vi "CLT_RunStateMach.vi"(6 "Test Index":i32, 7 "FullConfig":T6={"Bench Params"={"Relative Root Name"="", "Values"={"Step Levels"=0.0, "Resistor Tolerence"=0.0, "Sample Rate"=0.0, "Resistor"=0.0, "Wait Time"=0.0}, "Report Template path"=path "$ReportFiles/ReportTemplate_03.xlsx", "Test Type"="", "Config File Name"="", "Config 2 Use"="", "Skip Pre Lube"=FALSE}, "Test Params"=[], "Pump Params"={"Empty Inches"=0.0, "Full Inches"=0.0, "RNG_SLOW"=0.0, "RNG_CREEP"=0.0, "RNG_STOP "=0.0, "VISA resource name"="", "SPD_SLOW"=0, "SPD_CREEP"=0, "SPD_FAST"=0, "Zero template"=path "", "zero  Settle sec"=0, "Laser Slope"=0.0, "Laser Offset"=0.0, "Sim Fill Rate"=0.0, "Cal Date"="", "Cal Technician"=""}, "DataQ Params"={"Visa Name"="", "Num Chan"=0, "Cal Coef"=[], "Scale "=0, "Cal Date"="", "Cal Technicain"=""}, "Pump Control Ref"={"Fill "=refnum, "Drain"=refnum, "Level PV"=refnum, "Pump Speed"=refnum, "Run Test"=refnum, "Sim"=refnum, "Jog"=refnum, "Level SP"=refnum}, "Bench Status"={"Pump Status"=refnum, "Dataq Status"=refnum, "LaserStatus"=refnum, "ChA Ohms"=refnum, "ChB Ohms"=refnum}} {"Pump Params"."Sim Fill Rate" format="%.3f"; "Pump Params"."Laser Offset" format="%.3f"; "Pump Params"."Laser Slope" format="%.3f"; "Pump Params"."RNG_STOP" format="%#_13g"; "Pump Params"."RNG_CREEP" format="%#_13g"; "Pump Params"."RNG_SLOW" format="%#_13g"}, 11 "TEST State In":T5) -> (1 "Enable":bool, 2 "Level S":dbl, 3 "TEST State Out":T5, 4 "Test Index Out":i32, 5 "Specs Out":T1)   [LabVIEW 2024]
doc: "The \"Run Test\" button selects between MANUAL adjustment of Set Point (SP) by the user or AUTO mode, where:\n1. Start, initial state drains until the tank is empty\n2. Filling, Auto set of SP to Max Fill Inches (or recipie)\n3. FULL Pause when full\n4. Draining Auto set of SP to 0 (or recipie)\n5. EMPTY Paue when empty\n6. Done SP set to 0."
uses:
  Control Definitions/DEF_FullConfig.ctl
  Control Definitions/DEF_BenchParams.ctl
  Control Definitions/DEF_PumpParams.ctl
  Control Definitions/DEF_DataqParams.ctl
  Control Definitions/DEF_PumpCtlRefs.ctl
  Control Definitions/Def_PumpSpeed.ctl
  Control Definitions/DEF_BenchStatus.ctl
  Control Definitions/Def TestState.ctl
  Control Definitions/DEF_SpecsOut.ctl
  Control Definitions/Def Spec RNG.ctl
  Control Definitions/Ded LUT_Status.ctl
  Control Definitions/Global 2.vi
panel:
  out "Timer":dbl
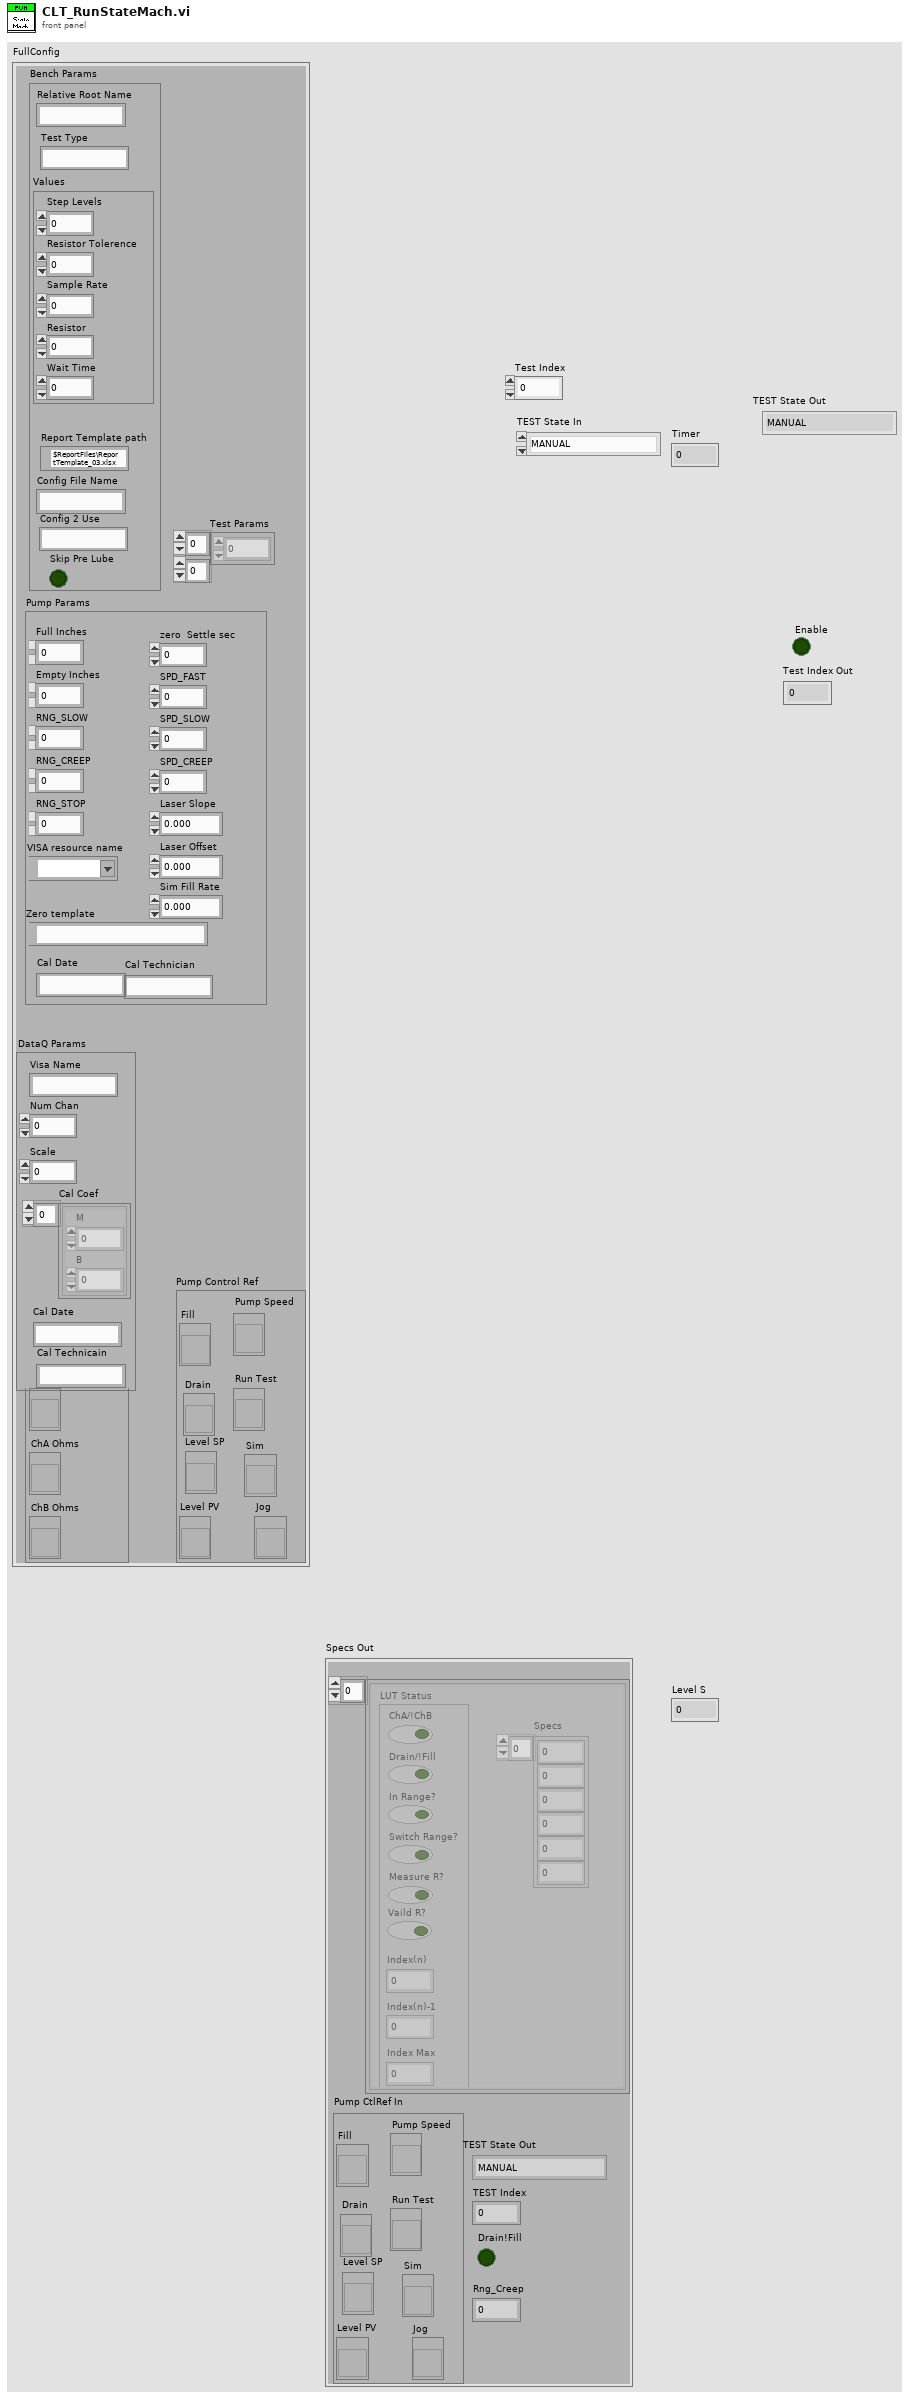
[diagram p1: front panel]
types:
  T1 = typedef "DEF_SpecsOut.ctl" = cluster{"aSpecsTable":T2[], "Pump CtlRef In":T4, "TEST State Out":T5, "TEST Index":i32, "Drain!Fill":bool, "Rng_Creep":dbl}
  T2 = typedef "Def Spec RNG.ctl" = cluster{"Specs":dbl[], "LUT Status":T3}
  T3 = typedef "Ded LUT_Status.ctl" = cluster{"ChA/!ChB":bool, "Drain/!Fill":bool, "In Range?":bool, "Switch Range?":bool, "Measure R?":bool, "Vaild R?":bool, "Index(n)":i32, "Index(n)-1":i32, "Index Max":i32, "Index(n-1)":i32}
  T4 = typedef "DEF_PumpCtlRefs.ctl" = cluster{"Fill ":refnum<vi>, "Drain":refnum<vi>, "Level PV":refnum<vi>, "Pump Speed":refnum<vi>, "Run Test":refnum<vi>, "Sim":refnum<vi>, "Jog":refnum<vi>, "Level SP":refnum<vi>}
  T5 = typedef "Def TestState.ctl" = enum16{"MANUAL", "Start", "Pre-Fill", "Pre-Fill Measure", "Pre-Drain", "Pre-Drain Measure", "Init-Record", "Load Fill Spec", "Filling Hi", "Wait1", "Record Fill", "Load Drain Spec", "Draining Lo", "Wait2", "Record Drain", "Empty", "Done"}
  T6 = typedef "DEF_FullConfig.ctl" = cluster{"Bench Params":T7, "Test Params":dbl[][], "Pump Params":T8, "DataQ Params":T9, "Pump Control Ref":T4, "Bench Status":T10}
  T7 = typedef "DEF_BenchParams.ctl" = cluster{"Relative Root Name":string, "Values":cluster{"Step Levels":dbl, "Resistor Tolerence":dbl, "Sample Rate":dbl, "Resistor":dbl, "Wait Time":dbl}, "Report Template path":path, "Test Type":string, "Config File Name":string, "Config 2 Use":string, "Skip Pre Lube":bool}
  T8 = typedef "DEF_PumpParams.ctl" = cluster{"Empty Inches":dbl, "Full Inches":dbl, "RNG_SLOW":dbl, "RNG_CREEP":dbl, "RNG_STOP ":dbl, "VISA resource name":refnum<visa-resource-name>, "SPD_SLOW":i32, "SPD_CREEP":i32, "SPD_FAST":i32, "Zero template":path, "zero  Settle sec":i32, "Laser Slope":sgl, "Laser Offset":sgl, "Sim Fill Rate":sgl, "Cal Date":string, "Cal Technician":string}
  T9 = typedef "DEF_DataqParams.ctl" = cluster{"Visa Name":string, "Num Chan":i32, "Cal Coef":cluster{"M":dbl, "B":dbl}[], "Scale ":i32, "Cal Date":string, "Cal Technicain":string}
  T10 = typedef "DEF_BenchStatus.ctl" = cluster{"Pump Status":refnum<vi>, "Dataq Status":refnum<vi>, "LaserStatus":refnum<vi>, "ChA Ohms":refnum<vi>, "ChB Ohms":refnum<vi>}
  T11 = typedef "Def_PumpSpeed.ctl" = enum16{"FAST", "SLOW", "CREEP", "STOP"}
  T12 = enum16{"MANUAL", "Start", "Filling", "FULL", "Draining", "EMPTY", "Done"}
  T13 = cluster{"Spec RNG Out":T2[], "Pump Control Ref":T4, "TEST State Out":u16, "Index":i32, bool, "RNG_CREEP":dbl}
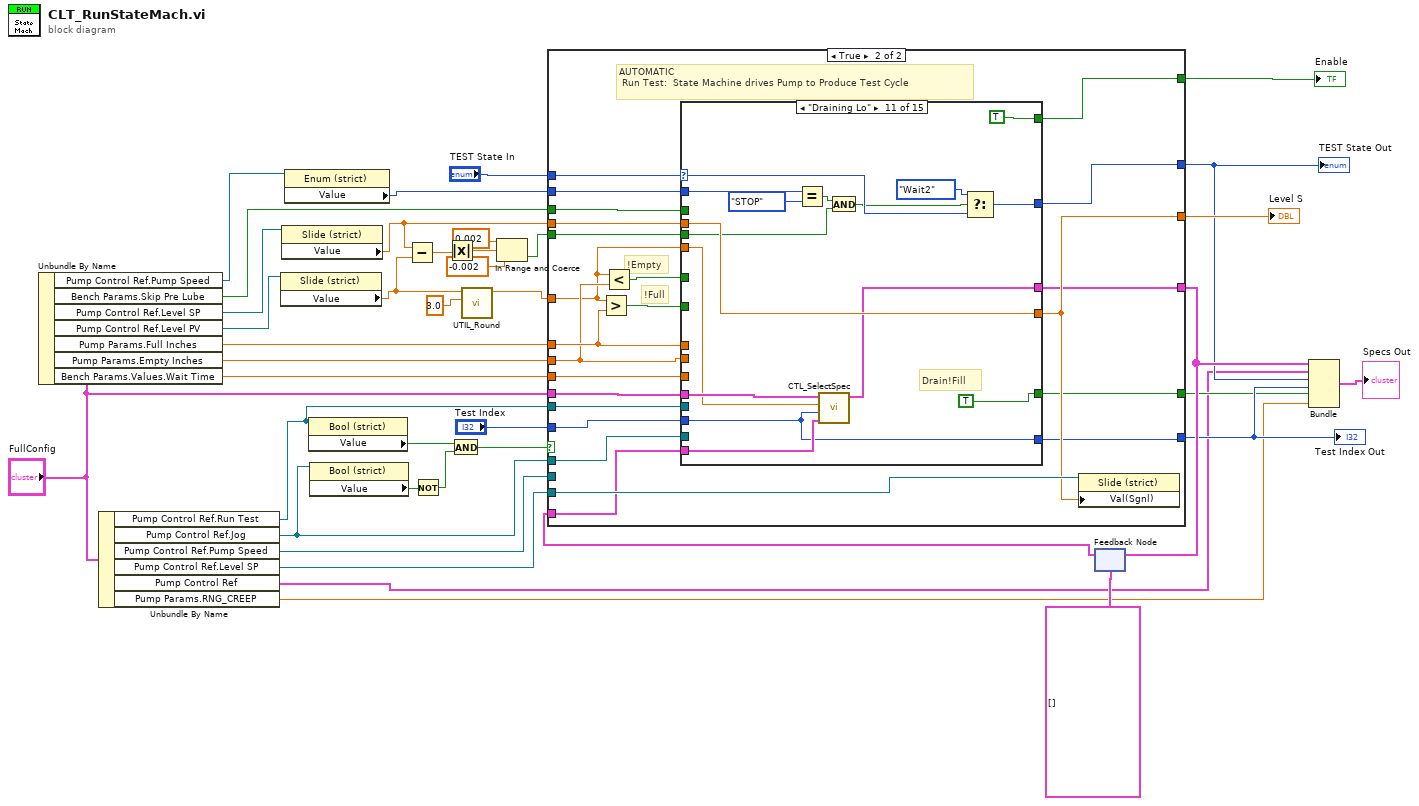
[diagram p0: block diagram]
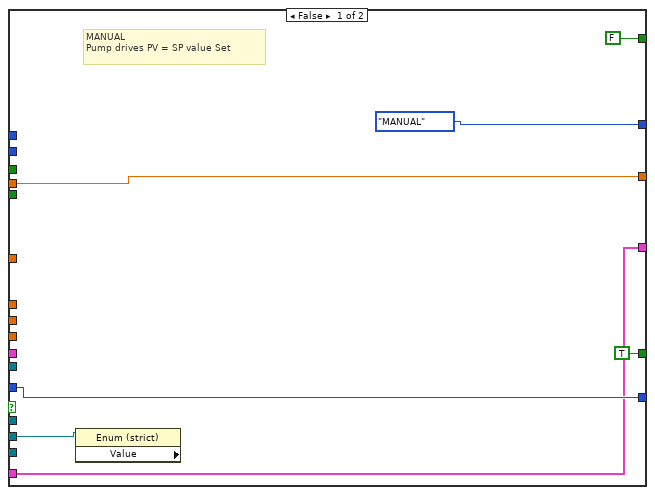
[diagram p2: hidden frame]
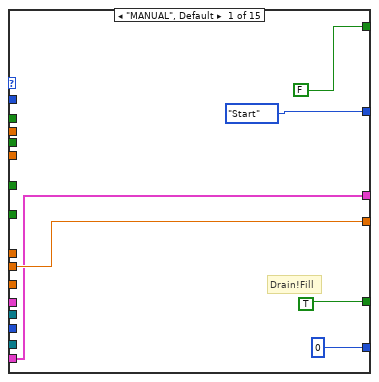
[diagram p3: hidden frame]
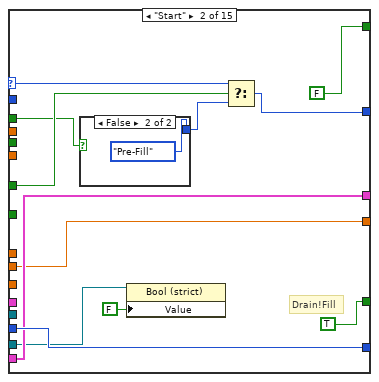
[diagram p4: hidden frame]
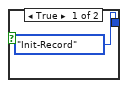
[diagram p5: hidden frame]
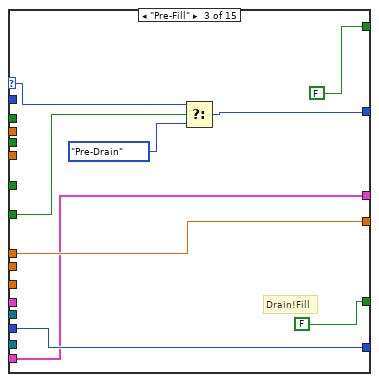
[diagram p6: hidden frame]
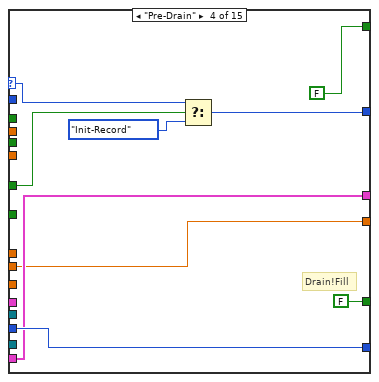
[diagram p7: hidden frame]
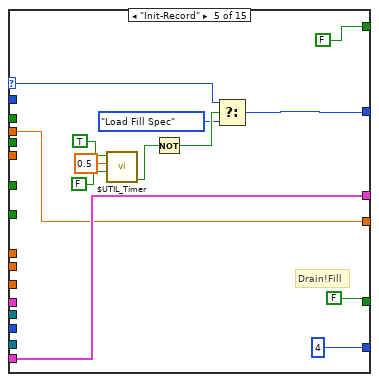
[diagram p8: hidden frame]
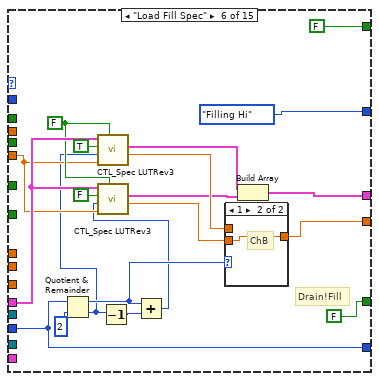
[diagram p9: hidden frame]
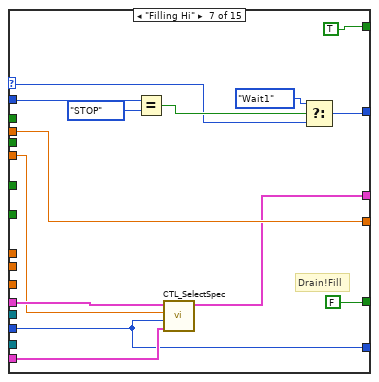
[diagram p11: hidden frame]
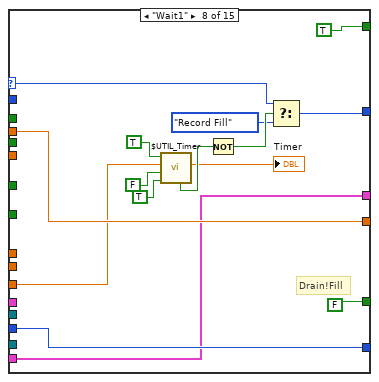
[diagram p12: hidden frame]
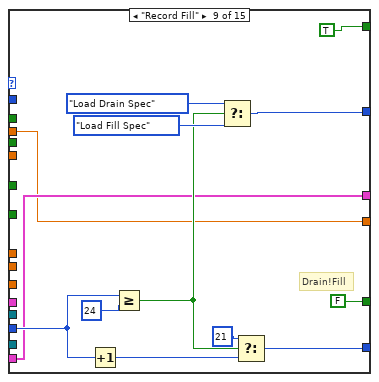
[diagram p13: hidden frame]
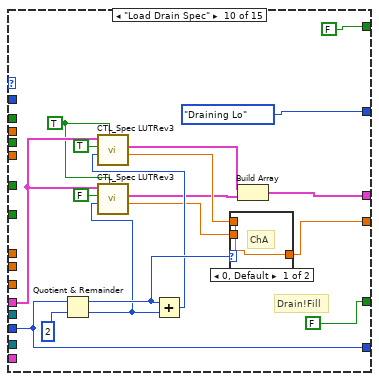
[diagram p14: hidden frame]
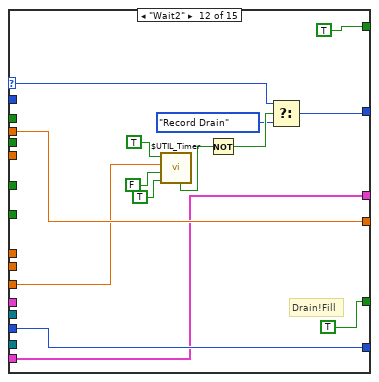
[diagram p16: hidden frame]
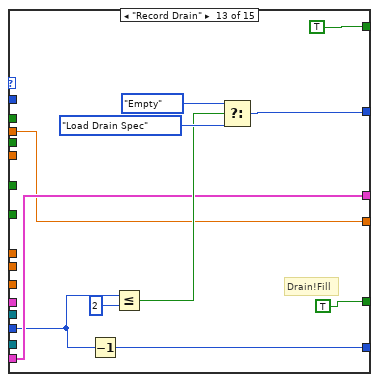
[diagram p17: hidden frame]
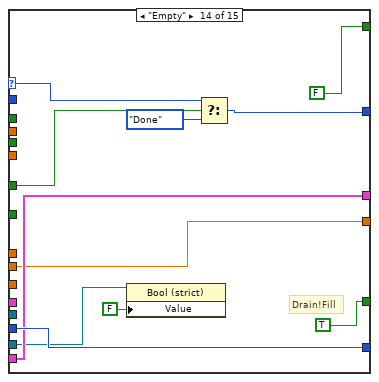
[diagram p18: hidden frame]
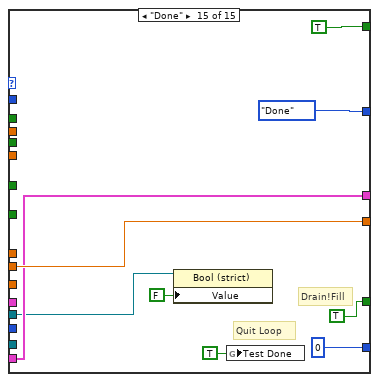
[diagram p19: hidden frame]
diagram:
  n1 = Unbundle By Name("FullConfig") -> ("Pump Control Ref.Pump Speed"=w18:refnum<vi>, "Bench Params.Skip Pre Lube"=w19:bool, "Pump Control Ref.Level SP"=w21:refnum<vi>, "Pump Control Ref.Level PV"=w20:refnum<vi>, "Pump Params.Full Inches"=w23:dbl, "Pump Params.Empty Inches"=w24:dbl, "Bench Params.Values.Wait Time"=w22:dbl)
  n2 = Unbundle By Name("FullConfig") -> ("Pump Control Ref.Run Test"=w14:refnum<vi>, "Pump Control Ref.Jog"=w5:refnum<vi>, "Pump Control Ref.Pump Speed"=w28:refnum<vi>, "Pump Control Ref.Level SP"=w27:refnum<vi>, "Pump Control Ref"=w26:T4, "Pump Params.RNG_CREEP"=w6:dbl)
  n3 = property class="Slide (strict)"(reference=w20) -> ("Value"=w12:dbl)  [unwired: 1 in, 2 out]
  n4 = property class="Slide (strict)"(reference=w21) -> ("Value"=w13:dbl)  [unwired: 1 in, 2 out]
  n5 = property class="Enum (strict)"(reference=w18) -> ("Value"=w17:T11)  [unwired: 1 in, 2 out]
  n6 = property class="Bool (strict)"(reference=w14) -> ("Value"=w2:bool)  [unwired: 1 in, 2 out]
  n7 = property class="Bool (strict)"(reference=w5) -> ("Value"=w4:bool)  [unwired: 1 in, 2 out]
  n8 = Subtract(x=w13, y=w12) -> (x-y=w11:dbl)
  n9 = Not(x=w4) -> (.not. x?=w3:bool)
  n10 = Absolute Value(x=w11) -> (abs(x)=w10:dbl)
  n11 = And(x=w2, y=w3) -> (x .and. y?=w1:bool)
  n12 = call "UTIL_Round.vi"("Significant decimal"=3.0 ("y"), "Number"=w12) -> ("Numeric"=w15:dbl)  [unwired: 9 in]
  n13 = In Range and Coerce(upper limit=0.002, x=w10, lower limit=-0.002) -> (In Range?=w7:bool)  [unwired: 1 out]
  n14 = feedback #1(T2[] []) -> (w35:T2[])
  n15 = case shown="True" w1 {
    tunnel: w13 -> [w45 w66]
    tunnel: "TEST State In" -> [_ w63]
    tunnel: w15 -> [_ w61]
    tunnel: [T12."MANUAL" ("TEST STATUS In in") w68] -> w30
    tunnel: w23 -> [_ w69]
    tunnel: w24 -> [_ w64]
    tunnel: w27 -> [_ w65]
    tunnel: [w45 w62] -> w37
    tunnel: "Test Index" -> [w44 w60]
    tunnel: "FullConfig" -> [_ w59]
    tunnel: [w44 w58] -> w31
    tunnel: [FALSE w57] -> w36
    tunnel: [w42 w56] -> w33
    tunnel: w35 -> [w42 w55]
    tunnel: w19 -> [_ w54]
    tunnel: w28 -> [w41 _]
    tunnel: w5 -> [_ w53]
    tunnel: [TRUE w52] -> w29
    tunnel: w22 -> [_ w51]
    tunnel: w17 -> [_ w50]
    tunnel: w14 -> [_ w48]
    tunnel: w7 -> [_ w47]
    frame False {
      # "MANUAL \nPump drives PV = SP value Set"
      n16 = property class="Enum (strict)" props=["Value"](reference=w41) -> ()  [unwired: 1 in, 3 out]
    }
    frame True {
      # "!Full"
      # "!Empty"
      # "AUTOMATIC\n Run Test:  State Machine drives Pump to Produce Test Cycle"
      n17 = Greater?(x=w61, y=w69) -> (0:w49:bool)
      n18 = Less?(x=w61, y=w64) -> (x < y?=w67:bool)
      n19 = case shown="\"Draining Lo\"" w63 {
        selector: w63 -> [_ w77 w91 w99 w113 _ w145 w169 _ _ w209 w232 _ w256 _]
        tunnel: w69 -> [_ _ w97 _ _ _ _ _ _ _ _ _ _ _ _]
        tunnel: [w75 w78 w97 w101 w108 w134 w156 w166 w172 w196 w219 w229 w235 w246 w265] -> w62
        tunnel: [Def_TestState."Start" ("TEST State Out") w87 w98 w107 w112 Def_TestState."Filling Hi" ("TEST State In") w143 w170 w183 Def_TestState."Draining Lo" ("TEST State In") w220 w233 w245 w255 Def_TestState."Done" ("TEST State Out")] -> w68
        tunnel: w67 -> [_ w86 _ w106 _ _ _ _ _ _ _ _ _ w254 _]
        tunnel: w49 -> [_ _ w96 _ _ _ _ _ _ _ _ _ _ _ _]
        tunnel: w64 -> [w75 w78 _ w101 _ _ _ _ _ _ _ _ _ w246 w265]
        tunnel: w66 -> [_ _ _ _ w108 _ w156 w166 w172 _ w219 w229 w235 _ _]
        tunnel: w61 -> [_ _ _ _ _ w124 w149 _ _ _ w212 _ _ _ _]
        tunnel: w60 -> [_ w85 w95 w105 _ w138 w151 w165 w180 w200 w213 w228 w237 w253 _]
        tunnel: w59 -> [_ _ _ _ _ w131 w150 _ _ w193 w214 _ _ _ _]
        tunnel: [0 ("Index") w85 w95 w105 4 ("Index") w138 w151 w165 w178 w200 w213 w228 w241 w253 0 ("Index")] -> w58
        tunnel: [FALSE FALSE FALSE FALSE FALSE FALSE TRUE TRUE TRUE FALSE TRUE TRUE TRUE FALSE TRUE] -> w57
        tunnel: [w71 w83 w93 w103 w110 w126 w153 w159 w174 w187 w215 w223 w239 w251 w260] -> w56
        tunnel: w55 -> [w71 w83 w93 w103 w110 _ w152 w159 w174 _ w216 w223 w239 w251 w260]
        tunnel: w54 -> [_ w82 _ _ _ _ _ _ _ _ _ _ _ _ _]
        tunnel: w53 -> [_ w81 _ _ _ _ _ _ _ _ _ _ _ w250 _]
        tunnel: [TRUE TRUE FALSE FALSE FALSE FALSE FALSE FALSE FALSE FALSE TRUE TRUE TRUE TRUE TRUE] -> w52
        tunnel: w51 -> [_ _ _ _ _ _ _ w157 _ _ _ w221 _ _ _]
        tunnel: w50 -> [_ _ _ _ _ _ w144 _ _ _ w211 _ _ _ _]
        tunnel: w48 -> [_ _ _ _ _ _ _ _ _ _ _ _ _ _ w258]
        tunnel: w47 -> [_ _ _ _ _ _ _ _ _ _ w205 _ _ _ _]
        frame "MANUAL", Default {
          # "Drain!Fill"
        }
        frame "Start" {
          # "Drain!Fill"
          n20 = case shown="False" w82 {
            tunnel: [Def_TestState."Init-Record" ("TEST State Out") Def_TestState."Pre-Fill" ("TEST State Out")] -> w76
            frame True {
            }
            frame False {
            }
          }
          n21 = property class="Bool (strict)"(reference=w81, "Value"=FALSE) -> ()  [unwired: 1 in, 2 out]
          n22 = Select(t=w77, s=w86, f=w76) -> (s? t:f=w87:T5)
        }
        frame "Pre-Fill" {
          # "Drain!Fill"
          n23 = Select(t=w91, s=w96, f=Def_TestState."Pre-Drain" ("TEST State In")) -> (s? t:f=w98:T5)
        }
        frame "Pre-Drain" {
          # "Drain!Fill"
          n24 = Select(t=w99, s=w106, f=Def_TestState."Init-Record") -> (s? t:f=w107:T5)
        }
        frame "Init-Record" {
          # "Drain!Fill"
          n25 = call "$UTIL_Timer.vi"("Reset"=FALSE, "Time (sec)"=0.5, "Start"=TRUE) -> ("Timed Out"=w111:bool)  [unwired: 3 in, 5 out]
          n26 = Not(x=w111) -> (.not. x?=w117:bool)
          n27 = Select(t=w113, s=w117, f=Def_TestState."Load Fill Spec") -> (s? t:f=w112:T5)
        }
        frame "Load Fill Spec" {
          w130 = FALSE ("Drain!Fill")
          # "Drain!Fill"
          n28 = Quotient & Remainder(x=w138, y=2) -> (x-y*floor(x/y)=w136:i32, floor(x/y)=w122:i32)
          n29 = call "CTL_Spec LUTRev3.vi"("Drain!Fill"=w130, "Level IN inches"=w124, "Index"=w122, "ChA/!ChB"=TRUE, "FullConfig"=w131) -> ("Set Point"=w135:dbl, "Spec Range Out"=w128:T2)  [unwired: 3 in, 2 out]
          n30 = Decrement(x=w122) -> (x-1=w123:i32)
          n31 = Add(x=w136, y=w123) -> (x+y=w121:i32)
          n32 = call "CTL_Spec LUTRev3.vi"("Drain!Fill"=w130, "Level IN inches"=w124, "Index"=w121, "ChA/!ChB"=FALSE, "FullConfig"=w131) -> ("Set Point"=w129:dbl, "Spec Range Out"=w127:T2)  [unwired: 3 in, 2 out]
          n33 = case shown="1" w136 {
            tunnel: w135 -> [w141 _]
            tunnel: [w141 w142] -> w134
            tunnel: w129 -> [_ w142]
            frame 0, Default {
              # "ChA"
            }
            frame 1 {
              # "ChB"
            }
          }
          n34 = Build Array(w128, w127) -> (w126:T2[])
        }
        frame "Filling Hi" {
          # "Drain!Fill"
          n35 = Equal?(x=w144, y=Def_PumpSpeed."STOP") -> (x = y?=w147:bool)
          n36 = call "CTL_SelectSpec.vi"("Spec RNG In"=w152, "Test Index"=w151, "Level"=w149, "FullConfig"=w150) -> ("Spec RNG Out"=w153:T2[])  [unwired: 7 in]
          n37 = Select(t=Def_TestState."Wait1" ("f"), s=w147, f=w145) -> (s? t:f=w143:T5)
        }
        frame "Wait1" {
          # "Drain!Fill"
          n38 = call "$UTIL_Timer.vi"("Auto Reset"=TRUE, "Reset"=FALSE, "Time (sec)"=w157, "Start"=TRUE) -> ("Numeric 2"=→"Timer":dbl, "TO Trig"=w161:bool)  [unwired: 2 in, 4 out]
          n39 = Not(x=w161) -> (.not. x?=w168:bool)
          n40 = Select(t=w169, s=w168, f=Def_TestState."Record Fill") -> (s? t:f=w170:T5)
        }
        frame "Record Fill" {
          # "Drain!Fill"
          n41 = Increment(x=w180) -> (x+1=w179:i32)
          n42 = Greater Or Equal?(x=w180, y=24) -> (x >= y?=w176:bool)
          n43 = Select(t=Def_TestState."Load Drain Spec", s=w176, f=Def_TestState."Load Fill Spec" ("TEST State Out")) -> (s? t:f=w183:T5)
          n44 = Select(t=21, s=w176, f=w179) -> (s? t:f=w178:i32)
        }
        frame "Load Drain Spec" {
          w192 = TRUE ("Drain!Fill")
          # "Drain!Fill"
          n45 = Quotient & Remainder(x=w200, y=2) -> (x-y*floor(x/y)=w198:i32, floor(x/y)=w185:i32)
          n46 = call "CTL_Spec LUTRev3.vi"("Drain!Fill"=w192, "Index"=w185, "ChA/!ChB"=FALSE, "FullConfig"=w193) -> ("Set Point"=w190:dbl, "Spec Range Out"=w188:T2)  [unwired: 4 in, 2 out]
          n47 = Add(x=w198, y=w185) -> (x+y=w191:i32)
          n48 = call "CTL_Spec LUTRev3.vi"("Drain!Fill"=w192, "Index"=w191, "ChA/!ChB"=TRUE, "FullConfig"=w193) -> ("Set Point"=w197:dbl, "Spec Range Out"=w189:T2)  [unwired: 4 in, 2 out]
          n49 = case shown="0, Default" w198 {
            tunnel: w197 -> [w203 _]
            tunnel: [w203 w204] -> w196
            tunnel: w190 -> [_ w204]
            frame 0, Default {
              # "ChA"
            }
            frame 1 {
              # "ChB"
            }
          }
          n50 = Build Array(w189, w188) -> (w187:T2[])
        }
        frame "Draining Lo" {
          # "Drain!Fill"
          n51 = Equal?(x=w211, y=Def_PumpSpeed."STOP") -> (x = y?=w207:bool)
          n52 = call "CTL_SelectSpec.vi"("Spec RNG In"=w216, "Test Index"=w213, "Level"=w212, "FullConfig"=w214) -> ("Spec RNG Out"=w215:T2[])  [unwired: 7 in]
          n53 = And(x=w207, y=w205) -> (x .and. y?=w206:bool)
          n54 = Select(t=Def_TestState."Wait2" ("f"), s=w206, f=w209) -> (s? t:f=w220:T5)
        }
        frame "Wait2" {
          # "Drain!Fill"
          n55 = call "$UTIL_Timer.vi"("Auto Reset"=TRUE, "Reset"=FALSE, "Time (sec)"=w221, "Start"=TRUE) -> ("TO Trig"=w224:bool)  [unwired: 2 in, 5 out]
          n56 = Not(x=w224) -> (.not. x?=w231:bool)
          n57 = Select(t=w232, s=w231, f=Def_TestState."Record Drain") -> (s? t:f=w233:T5)
        }
        frame "Record Drain" {
          # "Drain!Fill"
          n58 = Decrement(x=w237) -> (x-1=w241:i32)
          n59 = Less Or Equal?(x=w237, y=2) -> (x <= y?=w242:bool)
          n60 = Select(t=Def_TestState."Empty", s=w242, f=Def_TestState."Load Drain Spec" ("TEST State Out")) -> (s? t:f=w245:T5)
        }
        frame "Empty" {
          # "Drain!Fill"
          n61 = property class="Bool (strict)"(reference=w250, "Value"=FALSE) -> ()  [unwired: 1 in, 2 out]
          n62 = Select(t=w256, s=w254, f=Def_TestState."Done") -> (s? t:f=w255:T5)
        }
        frame "Done" {
          # "Drain!Fill"
          # "Quit Loop"
          n63 = property class="Bool (strict)"(reference=w258, "Value"=FALSE) -> ()  [unwired: 1 in, 2 out]
          n64 = global write "Global 2.vi" "Test Done"(TRUE ("Test Done")) -> ()
        }
      }
      n65 = property class="Slide (strict)"(reference=w65, "Val(Sgnl)"=w62) -> ()  [unwired: 1 in, 2 out]
    }
  }
  "Test Index Out" <- w31
  "TEST State Out" <- w30
  "Enable" <- w36
  "Level S" <- w37
  n66 = feedback-in #1(w33) -> ()
  n67 = Bundle("Spec RNG Out"=w33, "Pump Control Ref"=w26, "TEST State Out"=w30, "Index"=w31, w29, "RNG_CREEP"=w6) -> (→"Specs Out":T13)  [unwired: 1 in]
